vi "HV Stat Monitor.vi"() -> (0 "output array":string[][](array[string]), 3 "transposed array":string[][](array[string]))   [LabVIEW 2018, in "HV QMH.lvlib"]
uses:
  HV QMH.lvlib
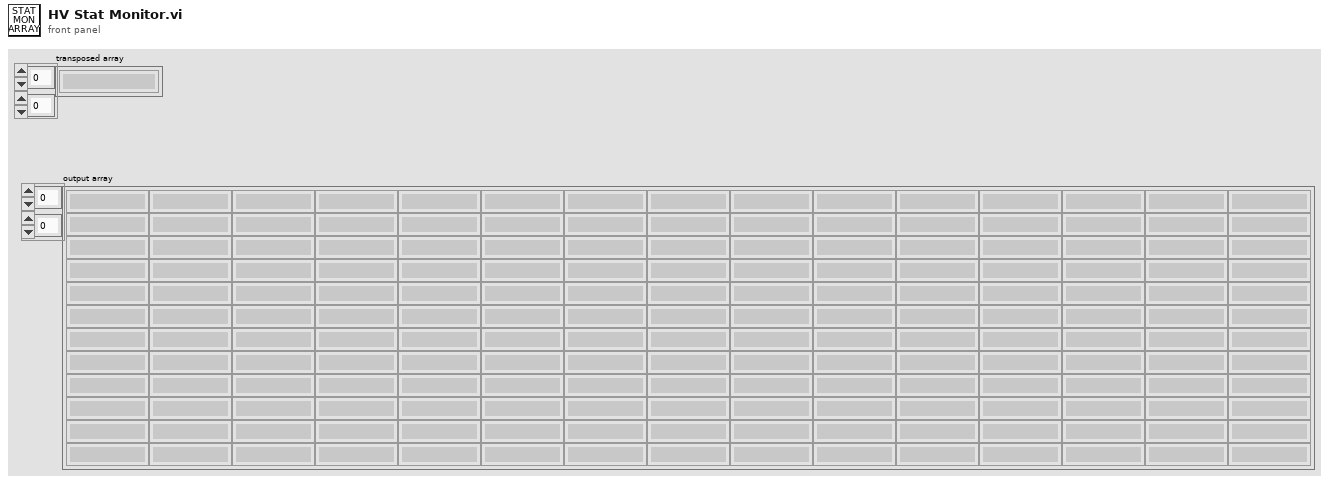
[diagram p1: front panel]
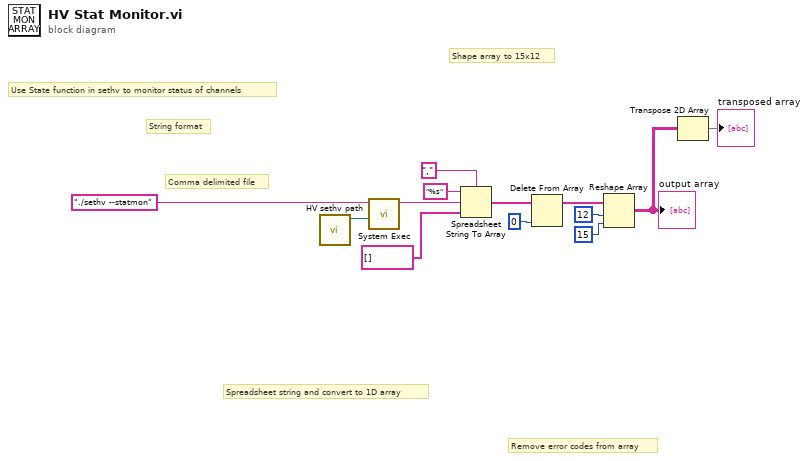
[diagram p0: block diagram]
diagram:
  # "String format"
  # "Comma delimited file"
  # "Shape array to 15x12"
  # "Remove error codes from array"
  # "Spreadsheet string and convert to 1D array"
  # "Use State function in sethv to monitor status of channels"
  n1 = call "HV sethv path.vi"() -> ("sethv filepath"=w13:path)  [unwired: 11 in]
  n2 = call <vilib>:"System Exec.vi"("working directory"=w13, "command line"="./sethv --statmon" ("string")) -> ("standard output"=w3:string)  [unwired: 6 in, 3 out]
  n3 = Spreadsheet String To Array(delimiter (Tab)=",", format string="%s", spreadsheet string=w3, array type (2D Dbl)=string[] []) -> (array=w7:string[])
  n4 = Delete From Array(array=w7, index=0) -> (array with subset deleted=w9:string[])  [unwired: 1 in, 1 out]
  n5 = Reshape Array(w9, 12 ("dimension size"), 15 ("dimension size")) -> (w12:string[][])
  "output array" <- w12
  n6 = Transpose 2D Array(2D array=w12) -> (transposed array=→"transposed array":string[][])
